vi "AutomatedTasks.vi"(8 "error in":errorcluster) -> ()   [LabVIEW 2014]
uses:
  <vilib>/Rock Robotics/WPI/Joystick/WPI_JoystickGetSetRefNum.vi
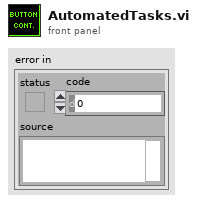
[diagram p1: front panel]
types:
  T1 = typedef "WPI_JoystickDevRef.ctl" = cluster{"Device":T2}
  T2 = typedef "WPI_JoystickDeviceEnum.ctl" = enum16{"USB 0", "USB 1", "USB 2", "USB 3", "USB 4", "USB 5"}
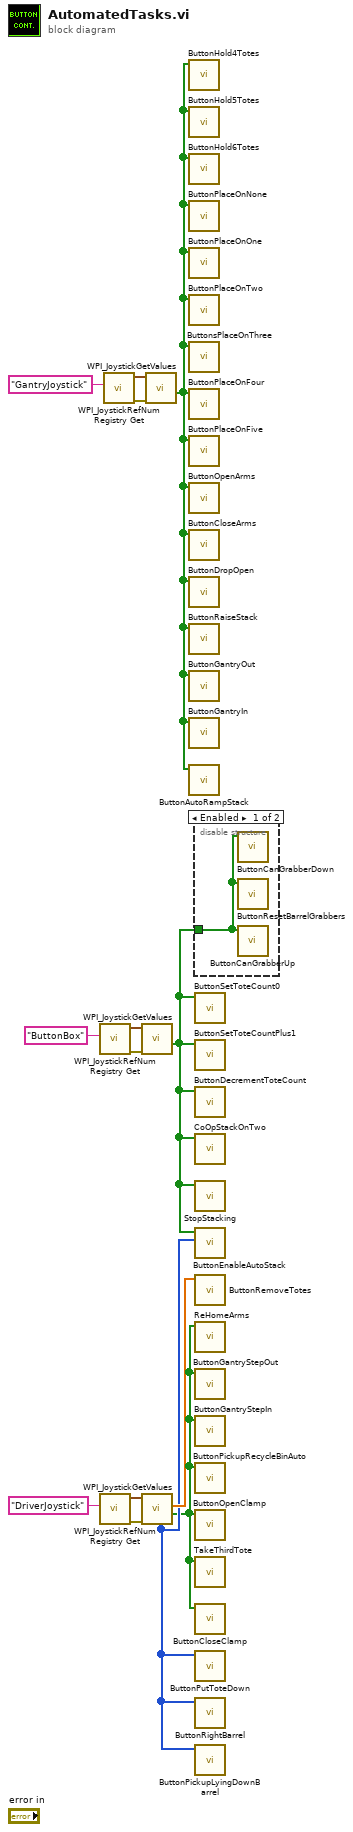
[diagram p0: block diagram]
diagram:
  n1 = call <vilib>:"WPI_JoystickRefNum Registry Get.vi"("refnum name"="ButtonBox") -> ("error out"=w5:errorcluster, "JoystickDevRef"=w6:T1)  [unwired: 9 in]
  n2 = call <vilib>:"WPI_JoystickRefNum Registry Get.vi"("refnum name"="DriverJoystick") -> ("error out"=w10:errorcluster, "JoystickDevRef"=w11:T1)  [unwired: 9 in]
  n3 = call <vilib>:"WPI_JoystickRefNum Registry Get.vi"("refnum name"="GantryJoystick") -> ("error out"=w13:errorcluster, "JoystickDevRef"=w14:T1)  [unwired: 9 in]
  n4 = call <vilib>:"WPI_JoystickGetValues.vi"("error in (no error)"=w5, "JoystickDevRef"=w6) -> ("Buttons"=w2:bool[])  [unwired: 5 in, 4 out]
  n5 = call <vilib>:"WPI_JoystickGetValues.vi"("error in (no error)"=w10, "JoystickDevRef"=w11) -> ("Buttons"=w1:bool[], "Axes"=w8:dbl[], "POVs"=w3:i16[])  [unwired: 5 in, 2 out]
  n6 = call <vilib>:"WPI_JoystickGetValues.vi"("error in (no error)"=w13, "JoystickDevRef"=w14) -> ("Buttons"=w7:bool[])  [unwired: 5 in, 4 out]
  n7 = call "ButtonHold4Totes.vi"("Buttons"=w7) -> ()  [unwired: 10 in, 1 out]
  n8 = call "ButtonHold5Totes.vi"("Buttons"=w7) -> ()  [unwired: 11 in]
  n9 = call "ButtonHold6Totes.vi"("Buttons"=w7) -> ()  [unwired: 11 in]
  n10 = call "ButtonPlaceOnNone.vi"("Buttons"=w7) -> ()  [unwired: 11 in]
  n11 = call "ButtonPlaceOnOne.vi"("Buttons"=w7) -> ()  [unwired: 11 in]
  n12 = call "ButtonPlaceOnTwo.vi"("Buttons"=w7) -> ()  [unwired: 11 in]
  n13 = call "ButtonsPlaceOnThree.vi"("Buttons"=w7) -> ()  [unwired: 11 in]
  n14 = call "ButtonPlaceOnFour.vi"("Buttons"=w7) -> ()  [unwired: 11 in]
  n15 = call "ButtonPlaceOnFive.vi"("Buttons"=w7) -> ()  [unwired: 11 in]
  n16 = call "ButtonOpenArms.vi"("Buttons"=w7) -> ()  [unwired: 11 in]
  n17 = call "ButtonCloseArms.vi"("Buttons"=w7) -> ()  [unwired: 11 in]
  n18 = call "ButtonDropOpen.vi"("Buttons"=w7) -> ()  [unwired: 10 in, 1 out]
  n19 = call "ButtonRaiseStack.vi"("Buttons"=w7) -> ()  [unwired: 11 in]
  n20 = call "ButtonGantryOut.vi"("Buttons"=w7) -> ()  [unwired: 11 in]
  n21 = call "ButtonGantryIn.vi"("Buttons"=w7) -> ()  [unwired: 11 in]
  n22 = call "ButtonAutoRampStack.vi"("Buttons"=w7) -> ()  [unwired: 11 in]
  n23 = disable-structure shown="Enabled" {
    disable-tunnel: w2 -> [w15 _]
    frame Enabled {
      n24 = call "ButtonCanGrabberDown.vi"("Buttons"=w15) -> ()  [unwired: 11 in]
      n25 = call "ButtonResetBarrelGrabbers.vi"("Buttons"=w15) -> ()  [unwired: 11 in]
      n26 = call "ButtonCanGrabberUp.vi"("Buttons"=w15) -> ()  [unwired: 11 in]
    }
    frame Disabled {
    }
  }
  n27 = call "ButtonSetToteCount0.vi"("Buttons"=w2) -> ()  [unwired: 11 in]
  n28 = call "ButtonSetToteCountPlus1.vi"("Buttons"=w2) -> ()  [unwired: 11 in]
  n29 = call "ButtonDecrementToteCount.vi"("Buttons"=w2) -> ()  [unwired: 11 in]
  n30 = call "CoOpStackOnTwo.vi"("Array"=w2) -> ()  [unwired: 11 in]
  n31 = call "StopStacking.vi"("Array"=w2) -> ()  [unwired: 11 in]
  n32 = call "ButtonEnableAutoStack.vi"("POVs"=w3, "Buttons"=w2) -> ()  [unwired: 10 in]
  n33 = call "ButtonRemoveTotes.vi"("array"=w8) -> ()  [unwired: 11 in]
  n34 = call "ReHomeArms.vi"("Array"=w1) -> ()  [unwired: 11 in]
  n35 = call "ButtonGantryStepOut.vi"("Buttons"=w1) -> ()  [unwired: 11 in]
  n36 = call "ButtonGantryStepIn.vi"("Buttons"=w1) -> ()  [unwired: 11 in]
  n37 = call "ButtonPickupRecycleBinAuto.vi"("Buttons"=w1) -> ()  [unwired: 10 in, 1 out]
  n38 = call "ButtonOpenClamp.vi"("Buttons"=w1) -> ()  [unwired: 11 in]
  n39 = call "TakeThirdTote.vi"("Array"=w1) -> ()  [unwired: 11 in]
  n40 = call "ButtonCloseClamp.vi"("Buttons"=w1) -> ()  [unwired: 11 in]
  n41 = call "ButtonPutToteDown.vi"("POVs"=w3) -> ()  [unwired: 11 in]
  n42 = call "ButtonRightBarrel.vi"("POVs"=w3) -> ()  [unwired: 11 in]
  n43 = call "ButtonPickupLyingDownBarrel.vi"("POVs"=w3) -> ()  [unwired: 11 in]
